vi "Agilent 428X Series Frequency Step Measurement .vi"(6 "Stop Freq (Hz)(1MHz)":dbl=1000000.0 min=20.0 max=30000000.0 step=10.0 format="%^.4e", 7 "Step Freq (Hz)(1KHz)":dbl=1000.0 min=0.0 max=30000000.0 step=10.0 format="%^.4e", 8 "error in (no error)":errorcluster, 9 "Start Freq (Hz)( 20 Hz)":dbl=20.0 min=20.0 max=30000000.0 step=10.0 format="%^.4e", 10 "Imp Type (0: CPD)":u32(ring) items=["CPD", "CPQ", "CPG", "CPRP", "CSD", "CSQ", "CSRS", "LPQ", "LPD", "LPG", "LPRP", "LSD", "LSQ", "LSRS", "RX", "ZTD", "ZTR", "GB", "YTD", "YTR"], 11 "VISA resource name":refnum<visa-resource-name>) -> (0 "error out":errorcluster, 1 "Primary Value":dbl format="%^.4e", 2 "Secondary Value":dbl format="%^.4e", 3 "VISA resource name out":refnum<visa-resource-name>, 4 "Data Status":bool=TRUE, 5 "?":cluster{dbl[], dbl[]}[](graph))   [LabVIEW 2015]
doc: "This VI is an example of how to use the HP428XA subVIs programmatically. This VI first configures a measurement, sets triggering, then takes measurements.\n\nThis function demonstrate one type of impedance measurement that can be made with the HP428XA and it accessories. In this example a 220 pF ceramic capacitor will be measured under the following conditions.\n\n DUT:\n 220 pF ceramic capacitor\n (HP Part Number 0160-4812)\n\n Measurement Conditions: \n \n Function: Cp-D\n Frequency: 1.0 MHz\n Test Signal Level: 1.0 V\n \n Equipment Required:\n\n HP 16047C Test Fixture\n Shorting bar (HP Part Number 5000-4226) or equivalent\n\nNote:\nFor more details see to the operation manual in Chapter 3."
uses:
  <instrlib>/Agilent 428X Series/Agilent 428X Series.lvlib
panel:
  # "© Copyright 2005 National Instruments Corporation.  All Rights Reserved."
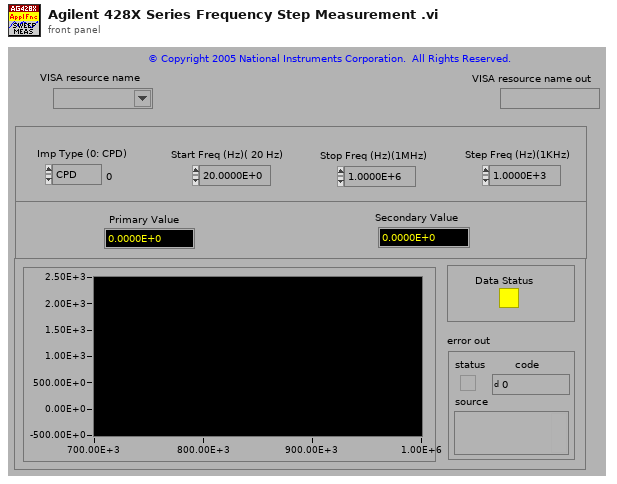
[diagram p1: front panel]
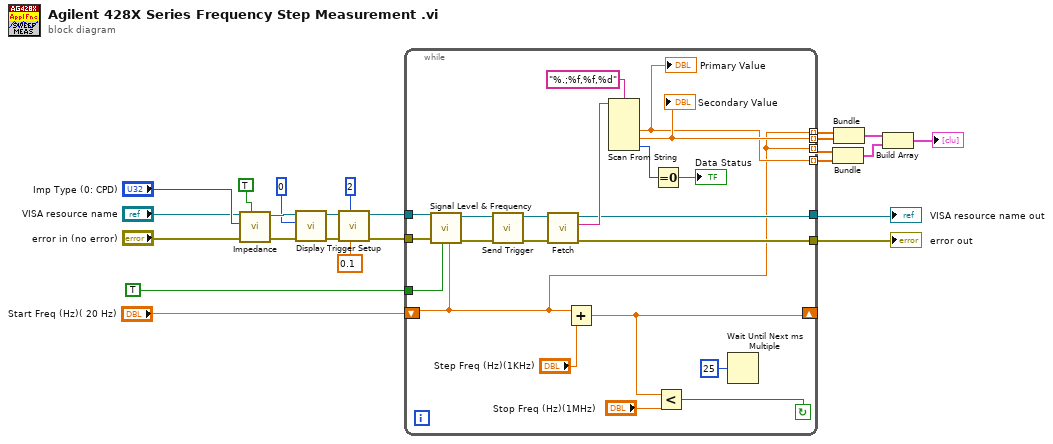
[diagram p0: block diagram]
diagram:
  n1 = call <instrlib>:"Impedance.vi"("Auto Range (F: Off)"=TRUE ("Auto Range (Off:F)"), "error in (no error)"="error in (no error)", "Imp Type (0: CPD)"="Imp Type (0: CPD)", "VISA resource name"="VISA resource name") -> ("error out"=w21:errorcluster, "VISA resource name out"=w24:refnum<visa-resource-name>)  [unwired: 6 in]
  n2 = call <instrlib>:"Display.vi"("error in (no error)"=w21, "Display Page (0: Measurement)"=u32 0 ("Display Page (Measurment:0)"), "VISA resource name"=w24) -> ("error out"=w22:errorcluster, "VISA resource name out"=w23:refnum<visa-resource-name>)  [unwired: 7 in]
  n3 = call <instrlib>:"Trigger Setup.vi"("Delay Value (s) (0.0)"=0.1, "Trigger Source (0: Internal)"=u32 2 ("Trigger Source (Internal:0)"), "error in (no error)"=w22, "VISA resource name"=w23) -> ("error out"=w11:errorcluster, "VISA resource name out"=w12:refnum<visa-resource-name>)  [unwired: 6 in]
  n4 = while {
    tunnel: [w26] -> w4 mode=indexing
    tunnel: [w28] -> w3 mode=indexing
    tunnel: [w26] -> w5 mode=indexing
    tunnel: [w27] -> w6 mode=indexing
    tunnel: TRUE ("Oscillator Select (T: Voltage)") -> [w34]
    tunnel: w11 -> [w32]
    tunnel: w12 -> [w33]
    shift-left: "Start Freq (Hz)( 20 Hz)" -> [w26]
    shift-right: [w29] -> _
    tunnel: [w40] -> w14
    tunnel: [w41] -> w15
    stop <- w38 continue-if-true
    n5 = call <instrlib>:"Signal Level & Frequency.vi"("Frequency Value (Hz) (100KHz)"=w26, "Oscillator Select (T: Voltage)"=w34, "error in (no error)"=w32, "VISA resource name"=w33) -> ("error out"=w31:errorcluster, "VISA resource name out"=w30:refnum<visa-resource-name>)  [unwired: 6 in]
    n6 = call <instrlib>:"Send Trigger.vi"("error in (no error)"=w31, "VISA resource name"=w30) -> ("error out"=w35:errorcluster, "VISA resource name out"=w36:refnum<visa-resource-name>)  [unwired: 8 in]
    n7 = call <instrlib>:"Fetch.vi"("error in (no error)"=w35, "VISA resource name"=w36) -> ("error out"=w40:errorcluster, "Returned Data"=w42:string, "VISA resource name out"=w41:refnum<visa-resource-name>)  [unwired: 7 in]
    n8 = Add(x=w26, y="Step Freq (Hz)(1KHz)") -> (x+y=w29:dbl)
    n9 = Scan From String(format string="%.;%f,%f,%d", input string=w42) -> (output 1=w27:dbl, output 2=w28:dbl, output 3=w44:i32)  [unwired: 5 in, 3 out]
    "Primary Value" <- w27
    "Secondary Value" <- w28
    n10 = Equal To 0?(x=w44) -> (x = 0?=→"Data Status":bool)
    n11 = Less?(x=w29, y="Stop Freq (Hz)(1MHz)") -> (x < y?=w38:bool)
    n12 = Wait Until Next ms Multiple(millisecond multiple=u32 25) -> ()  [unwired: 1 out]
  }
  "VISA resource name out" <- w15
  "error out" <- w14
  n13 = Bundle(w5, w6) -> (w7:cluster{dbl[], dbl[]})  [unwired: 1 in]
  n14 = Bundle(w4, w3) -> (w2:cluster{dbl[], dbl[]})  [unwired: 1 in]
  n15 = Build Array(w2, w7) -> (→"?":cluster{dbl[], dbl[]}[])
